vi "Fix-Bild laden.vi"(8 "error in (no error)":errorcluster caption="Fehler (Eingang, kein Fehler)", 11 "TDMS-Datei":refnum<k34>) -> (0 "error out":errorcluster caption="Fehler (Ausgang)", 2 "Fixbild":T1[](array[typedef]), 3 "TDMS-Datei (Ausgang)":refnum<k34>)   [LabVIEW 2020, in "Anlagenuebersicht.lvlib" / "VisBx Anzeige.lvlib" / "TDMS laden.lvlib"]
doc: "Liest die für den Aufbau eines Fixbildes benötigten Zeichenbefehle mit den zugehörigen Parametern aus einer bereits geöffneten TDMS-Datei. Die Daten werden nur für das Editieren (VisBx-Editor) gebraucht, nicht aber für die Anzeige der Visualisierung."
uses:
  TDMS laden.lvlib
  VisParameter/VisSchritt.ctl
  VisParameter/VisSchritt-Typ.ctl
  VisParameter/VisParam-Typdef.lvlib
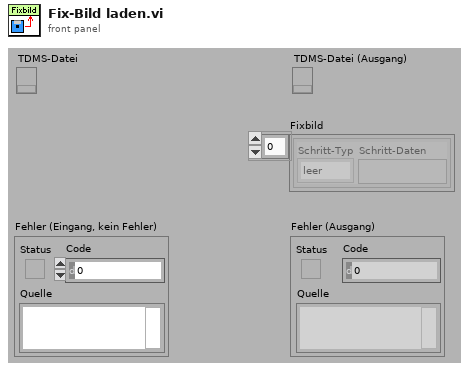
[diagram p1: front panel]
types:
  T1 = typedef "VisParam-Typdef.lvlib/VisSchritt.ctl" = cluster{"Schritt-Typ":T2, "Schritt-Daten":variant}
  T2 = typedef "VisParam-Typdef.lvlib/VisSchritt-Typ.ctl" = enum16{"leer", "Punkt", "Linie", "Linienzug", "Fixtext", "Textrechteck", "Ziffernanzeige", "Rechteck", "Rechteck rund", "Ellipse", "Bogen", "Kreis", "Pixmap"}
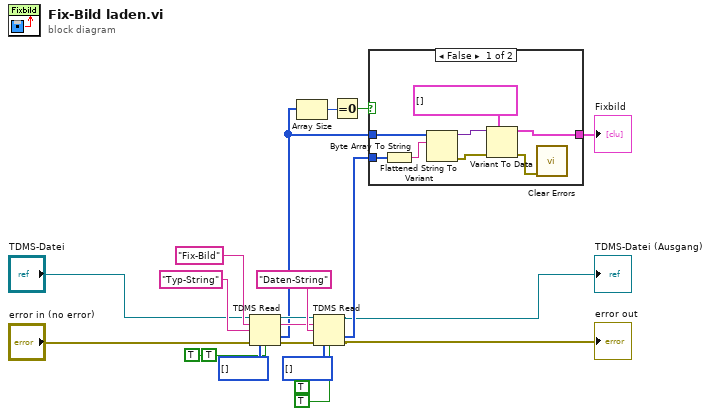
[diagram p0: block diagram]
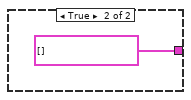
[diagram p2: hidden frame]
diagram:
  (unwired) TRUE ("Kanalreihenfolge von Datei beibehalten? (F)")
  (unwired) TRUE ("Kanalreihenfolge von Datei beibehalten? (F)")
  n1 = TDMS Read(0:"TDMS-Datei", 5:"Fix-Bild" ("Gruppenname (Eingang, Unbenannt)"), 7:"Typ-String" ("Kanalnamen (Eingang) (Unbenannt)"), 11:"error in (no error)", 12:i16[] [] ("Typ-String"), 13:TRUE ("Kanalreihenfolge von Datei beibehalten? (F)")) -> (4:w15:refnum<k34>, 6:w12:string, 10:w10:i16[], 15:w4:errorcluster)  [unwired: 2 in, 2 out]
  n2 = Array Size(array=w10) -> (size(s)=w8:i32)
  n3 = TDMS Read(0:w15, 5:w12, 7:"Daten-String" ("Kanalnamen (Eingang) (Unbenannt)"), 11:w4, 12:u8[] [] ("Vorzeichenloses Byte-Array"), 13:TRUE ("Kanalreihenfolge von Datei beibehalten? (F)")) -> (4:→"TDMS-Datei (Ausgang)":refnum<k34>, 10:w11:u8[], 15:→"error out":errorcluster)  [unwired: 2 in, 3 out]
  n4 = Equal To 0?(x=w8) -> (x = 0?=w9:bool)
  n5 = case shown="False" w9 {
    tunnel: [w27 T1[] [] ("Programm (Typ)")] -> w19
    tunnel: w11 -> [w24 _]
    tunnel: w10 -> [w22 _]
    frame False {
      n6 = Byte Array To String(unsigned byte array=w24) -> (string=w25:string)
      n7 = Flattened String To Variant(6:w25, 7:w22) -> (0:w21:errorcluster, 3:w26:variant)  [unwired: 1 in]
      n8 = Variant To Data(error in=w21, type=T1[] [] ("Programm (Typ)"), Variant=w26) -> (data=w27:T1[], error out=w20:errorcluster)
      n9 = call <vilib>:"Clear Errors.vi"("error in (no error)"=w20) -> ()  [unwired: 5 in, 2 out]
    }
    frame True {
    }
  }
  "Fixbild" <- w19
